vi "Result Status.vi"(9 "index no":i32, 11 "IL Sensor":bool[](array[boolean])) -> ()   [LabVIEW 2015]
uses:
  Galobal variable_TI.vi
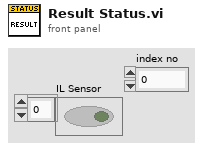
[diagram p1: front panel]
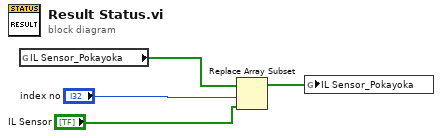
[diagram p0: block diagram]
diagram:
  n1 = global read "Galobal variable_TI.vi" "IL Sensor_Pokayoka"() -> (w3:bool[])
  n2 = Replace Array Subset(array=w3, new element="IL Sensor", index="index no") -> (w1:bool[])
  n3 = global write "Galobal variable_TI.vi" "IL Sensor_Pokayoka"(w1) -> ()
